vi "Robot Global Data.vi"() -> ()   [LabVIEW 2012]
doc: "This global VI can contain as many global variables as you need. Place a control on the panel, give it a good name. To read or write to it from a VI, drag the icon to the diagram of that VI. You can also drag from the project. Click on the node to change which global you access. You shouldn't have multiple locations writing to a global or it will cause a race-condition."
uses:
  <vilib>/Rock Robotics/WPI/Camera/WPI_CameraImageSize.ctl
  <vilib>/Rock Robotics/WPI/DriverStation/WPI_DriverStationRobotMode2.ctl
panel:
  out "Frisbee Cam On":bool
  out "Frisbee PID On":bool
  out "Frisbee Shooter On":bool
  out "Frisbee Vision On":bool
  out "Frisbee Feeder Station":bool
  in  "Shoot Y Hat":dbl
  in  "Minimum RPM":dbl
  in  "Upper LED":bool
  in  "Lower LED":bool
  in  "Shoot Button 10":bool
  in  "Insight Loop Count":dbl
  in  "Shooter RPM":dbl
  in  "Right Drive Button 8":bool
  in  "Right Drive Button 7":bool
  in  "Right Drive Button 6":bool
  in  "Right Drive Button 5":bool
  in  "Right Drive Button 4":bool
  in  "Right Drive Button 3":bool
  in  "Right Drive Button 2":bool
  in  "Right Drive Button 1":bool
  in  "High Y":dbl
  in  "Drive Button 8":bool
  in  "Drive Button 7":bool
  in  "Drive Button 6":bool
  in  "Drive Button 5":bool
  in  "Drive Button 4":bool
  in  "Drive Button 3":bool
  in  "Drive Button 2":bool
  in  "Vision Locked On":bool
  in  "Vision Offset":dbl
  in  "Shooter Vision Input":dbl
  out "Climb Override?":bool
  out "Vision Override?":bool
  out "Manual Override?":bool
  out "Shooter Full? T/F":bool
  in  "Shoot Twist Axis":dbl
  in  "Shoot Button 8":bool
  in  "Shoot Button 7":bool
  in  "Shoot Button 6":bool
  in  "Shoot Button 5":bool
  in  "Shoot Button 4":bool
  in  "Shoot Button 3":bool
  in  "Shoot Button 2":bool
  in  "Shoot X Axis":dbl
  in  "Shoot Y Axis":dbl
  in  "R Drive Y Axis":dbl
  in  "R Drive X Axis":dbl
  in  "L Drive Y Axis":dbl
  in  "L Drive X Axis":dbl
  in  "Shoot Button 1":bool
  in  "Drive Button 1":bool
  out "Shooter Empty? T/F":bool
  in  "Shooter Setpoint":dbl
  in  "Shooter Rotation Angle":dbl
  in  "Drivetrain Mode":dbl
  in  "Drive Mode":u16(ring) items=["Shooter Down"=1, "Shooter Up"=2]
  in  "Robot Mode":T1
  in  "LED toggle rate (ms)":u32=20
  in  "image size":T2=enum."320x240"
  in  "Enable Vision":bool
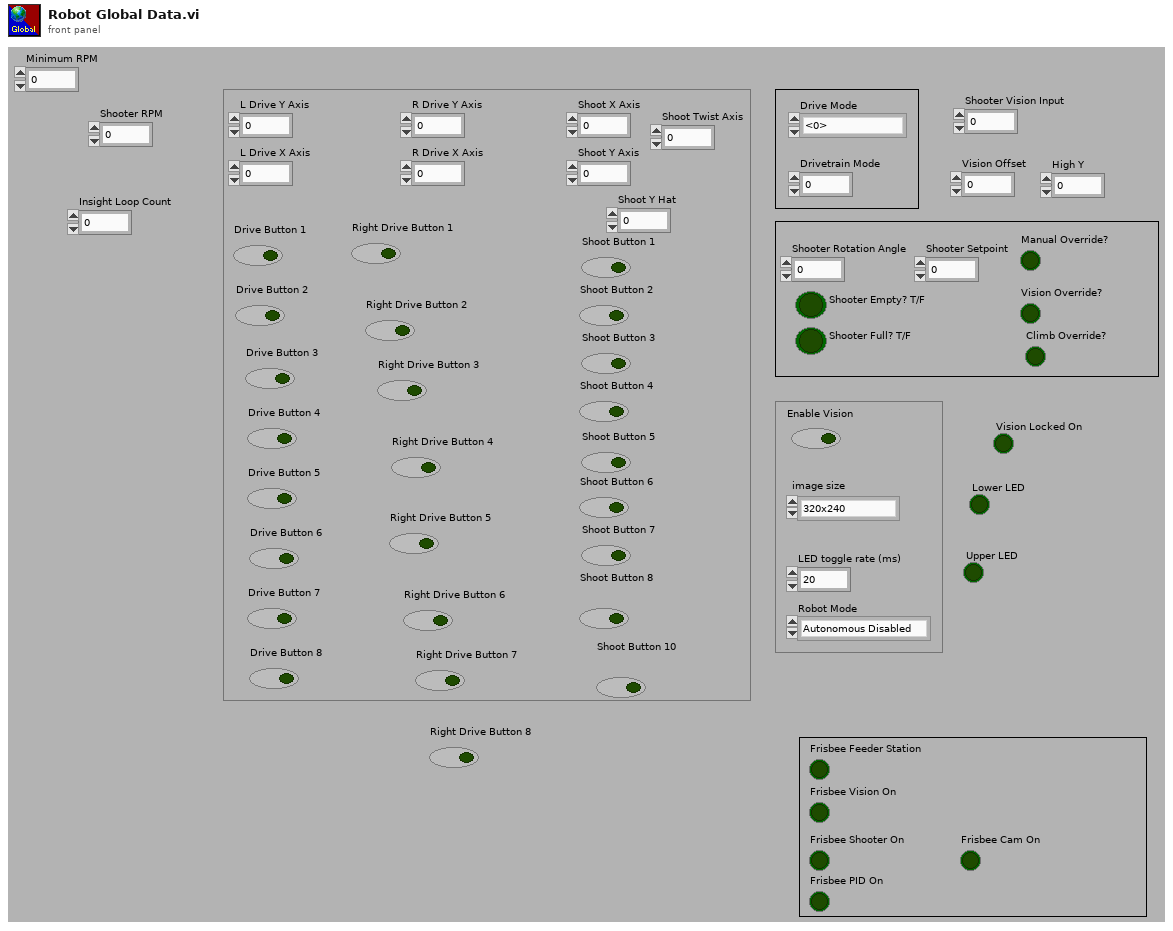
[diagram p1: front panel]
types:
  T1 = typedef "WPI_DriverStationRobotMode2.ctl" = enum16{"Autonomous Disabled", "Autonomous Enabled", "Teleop Disabled", "Teleop Enabled", "Timeout", "Finish", "Test Disabled", "Test Enabled"}
  T2 = typedef "WPI_CameraImageSize.ctl" = enum16{"640x480", "320x240", "160x120"}
diagram:
